vi "SubVI_Extract&Mask_RGB #.vi"(7 "Image Register Name":string="untitled", 8 "Error in":errorcluster, 10 "ROI Descriptor":T1 {"Contours"."Type" items=["No Selection", "Point", "Line", "Rectangle", "Oval", "Polygon", "Freehand Region", "Annulus", "Unused2", "Unused3", "Broken Line", "Freehand Line", "Rotated Rectangle"]}, 11 "Image Src In":T2) -> (0 "Error out":errorcluster, 1 "ROI Descriptor out":T1 {"Contours"."Type" items=["No Selection", "Point", "Line", "Rectangle", "Oval", "Polygon", "Freehand Region", "Annulus", "Unused2", "Unused3", "Broken Line", "Freehand Line", "Rotated Rectangle"]}, 2 "Image Dst Out":T2, 3 "Image Src Out":T2)   [LabVIEW 2013]
uses:
  <vilib>/vision/Image Controls.llb/IMAQ Image.ctl
  <vilib>/vision/NI_Vision_Development_Module.lvlib
panel:
  in  "Type":enum16{"Normal", "Exclude 0"}(ring)
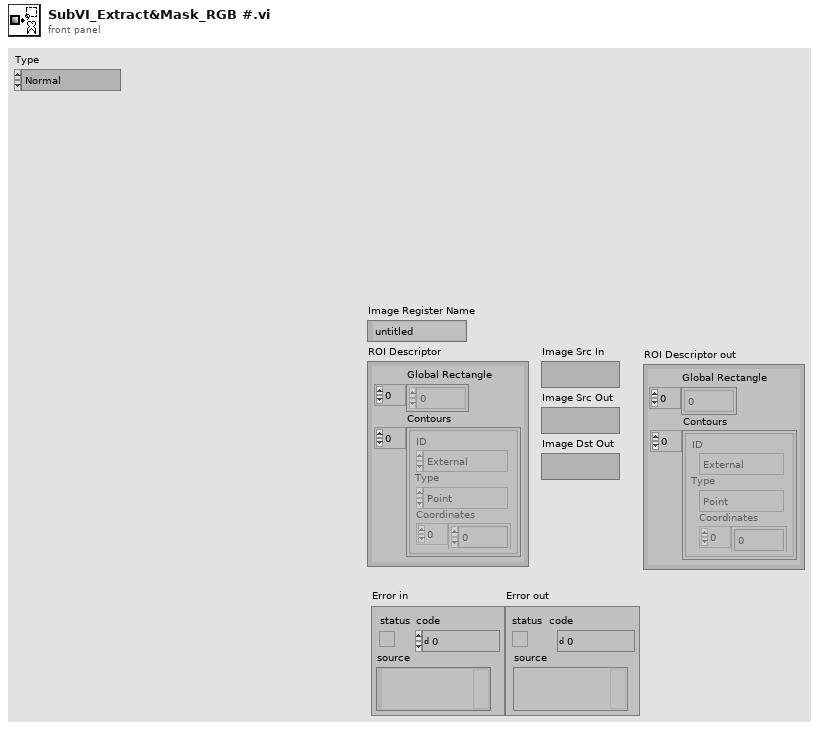
[diagram p1: front panel]
types:
  T1 = typedef "ROI Descriptor" = cluster{"Global Rectangle":i32[], "Contours":cluster{"ID":enum32{"External", "Internal"}, "Type":u32, "Coordinates":i32[]}[]}
  T2 = typedef "IMAQ Image.ctl" = refnum<image>
  T3 = typedef "Image Type" = u32
  T4 = cluster{"Origin":cluster{"X":sgl, "Y":sgl}, "Angle (deg)":sgl, "Axis Reference":u32}
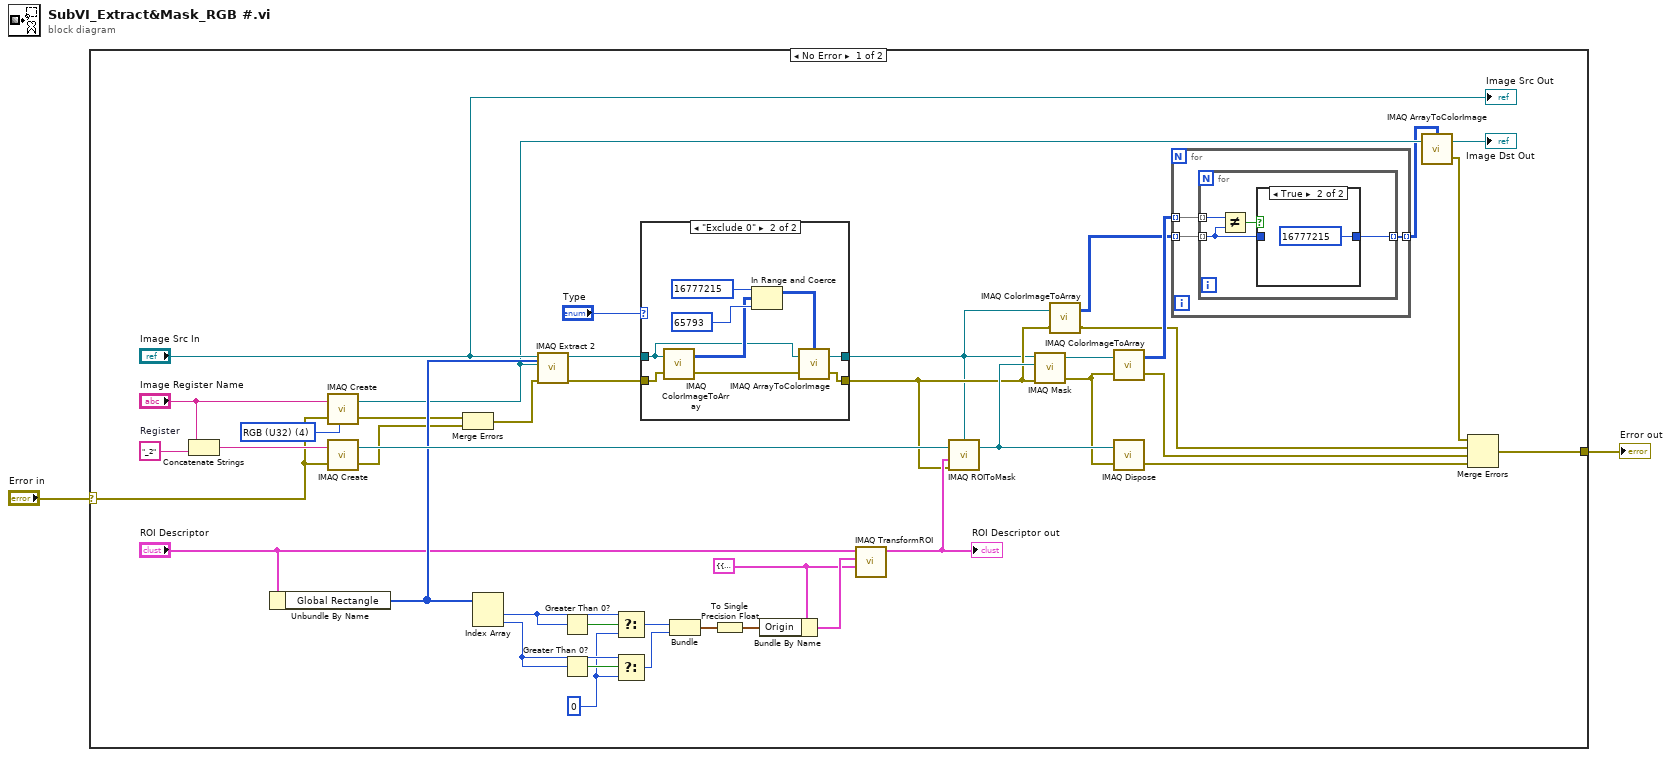
[diagram p0: block diagram]
diagram:
  n1 = case shown="No Error" "Error in" {
    selector: "Error in" -> [w21 w65]
    tunnel: [w33 w65] -> w2
    frame No Error {
      w20 = T3 4 items=["Grayscale (U8)", "Grayscale (I16)", "Grayscale (SGL)", "Complex (CSG)", "RGB (U32)", "HSL (U32)", "RGB (U64)", "Grayscale (U16)"] ("Image Type")
      w25 = 0
      w28 = T4 {"Origin"={"X"=0.0, "Y"=0.0}, "Angle (deg)"=0.0, "Axis Reference"=0} ("Base Reference")
      w40 = "_2"  # Register
      n2 = Concatenate Strings("Image Register Name", w40) -> (w42:string)
      n3 = Unbundle By Name("ROI Descriptor") -> ("Global Rectangle"=w39:i32[])
      n4 = call "IMAQ Create"("Image Name"="Image Register Name", "Image Type"=w20, "error in (no error)"=w21) -> ("New Image"=w12:T2, "error out"=w35:errorcluster)  [unwired: 2 in]
      n5 = call "IMAQ Create"("Image Name"=w42, "error in (no error)"=w21) -> ("New Image"=w44:T2, "error out"=w8:errorcluster)  [unwired: 3 in]
      n6 = Merge Errors(w35, w8) -> (w9:errorcluster)
      n7 = Index Array(array=w39) -> (element #1=w32:i32, element #2=w31:i32)  [unwired: 2 in]
      n8 = call "IMAQ Extract 2"("Optional Rectangle"=w39, "error in (no error)"=w9, "Image Dst"=w12, "Image Src"="Image Src In") -> ("error out"=w5:errorcluster, "Image Dst Out"=w6:T2)  [unwired: 6 in]
      n9 = Greater Than 0?(x=w32) -> (x > 0?=w27:bool)
      n10 = Greater Than 0?(x=w31) -> (x > 0?=w26:bool)
      n11 = Select(t=w32, s=w27, f=w25) -> (s? t:f=w24:i32)
      n12 = Select(t=w31, s=w26, f=w25) -> (s? t:f=w23:i32)
      n13 = case shown="\"Exclude 0\"" "Type" {
        tunnel: w5 -> [w45 w53]
        tunnel: [w45 w50] -> w4
        tunnel: [w46 w49] -> w3
        tunnel: w6 -> [w46 w47]
        frame "Normal", Default {
        }
        frame "Exclude 0" {
          n14 = call "IMAQ ColorImageToArray"("Image"=w47, "error in (no error)"=w53) -> ("Image Pixels (U32)"=w52:u32[][], "error out"=w51:errorcluster)  [unwired: 2 in, 1 out]
          n15 = In Range and Coerce(upper limit=u32 16777215, x=w52, lower limit=u32 65793) -> (coerced(x)=w48:u32[][])  [unwired: 1 out]
          n16 = call "IMAQ ArrayToColorImage"("Image Pixels (U32)"=w48, "Image"=w47, "error in (no error)"=w51) -> ("Image Out"=w49:T2, "error out"=w50:errorcluster)  [unwired: 2 in]
        }
      }
      n17 = Bundle(w24, w23) -> (w22:cluster{i32, i32})  [unwired: 1 in]
      n18 = To Single Precision Float(number=w22) -> (single precision float=w30:cluster{sgl, sgl})
      n19 = Bundle By Name(cluster=w28, "Origin"=w30) -> (w29:T4)
      n20 = call "IMAQ TransformROI"("New Reference"=w28, "Base Reference"=w29, "ROI Descriptor"="ROI Descriptor") -> ("ROI Descriptor out"=w37:T1)  [unwired: 7 in, 1 out]
      "ROI Descriptor out" <- w37
      n21 = call "IMAQ ROIToMask"("error in (no error)"=w4, "ROI Descriptor"=w37, "Image"=w44, "Image Model"=w3) -> ("Image Out"=w43:T2)  [unwired: 1 in, 3 out]
      n22 = call "IMAQ Mask"("error in (no error)"=w4, "Image Mask"=w43, "Image Src"=w3) -> ("error out"=w17:errorcluster, "Image Dst Out"=w19:T2)  [unwired: 1 in, 1 out]
      n23 = call "IMAQ ColorImageToArray"("Image"=w3, "error in (no error)"=w4) -> ("Image Pixels (U32)"=w14:u32[][], "error out"=w15:errorcluster)  [unwired: 2 in, 1 out]
      n24 = call "IMAQ ColorImageToArray"("Image"=w19, "error in (no error)"=w17) -> ("Image Pixels (U32)"=w16:u32[][], "error out"=w18:errorcluster)  [unwired: 2 in, 1 out]
      n25 = call "IMAQ Dispose"("Image"=w43, "error in (no error)"=w17) -> ("error out"=w34:errorcluster)  [unwired: 4 in]
      n26 = for {
        tunnel: w14 -> [w56] mode=indexing
        tunnel: w16 -> [w58] mode=indexing
        tunnel: [w57] -> w10 mode=indexing
        n27 = for {
          tunnel: w58 -> [w62] mode=indexing
          tunnel: [w60] -> w57 mode=indexing
          tunnel: w56 -> [w59] mode=indexing
          n28 = Not Equal?(x=w62, y=w59) -> (x != y?=w61:bool)
          n29 = case shown="True" w61 {
            tunnel: [w63 u32 16777215] -> w60
            tunnel: w59 -> [w63 _]
            frame False {
            }
            frame True {
            }
          }
        }
      }
      n30 = call "IMAQ ArrayToColorImage"("Image Pixels (U32)"=w10, "Image"=w12) -> ("Image Out"=→"Image Dst Out":T2, "error out"=w11:errorcluster)  [unwired: 3 in]
      n31 = Merge Errors(w11, w15, w18, w34) -> (w33:errorcluster)
      "Image Src Out" <- "Image Src In"
    }
    frame Error {
    }
  }
  "Error out" <- w2
